vi "Day 9-2.vi"() -> ()   [LabVIEW 2019, in "Day 9.lvlib"]
uses:
  Day 9.lvlib
panel:
  out "result":i32
  out "Array 4":i32[](array[numeric])
  out "logical OR":bool
  out "Array 3":i32[][](array[numeric])
  out "x = y?":bool[][](array[boolean])
  out "Array":i32[][](array[numeric])
  in  "String":string="8969799987646798965432975435334567987976999867976794468999979759865767896545699865678952123899325456\n7658678998434597654321984320123458976765789998965432367998968998754556789434987654489543535698912349\n6243457899325679997620195431934569765654667999993101246796856997643245679759865443356954656987894498\n4102345678912998789531297659895978954213456899874512659965239876432134578998754321267899877976789987\n3212466989109887678942989797659799542102345798765423867894103987543026799989866532345678999765469896\n43234878932997954898999789879476896542434967898768649889432124986541359999679877654667899876543..."
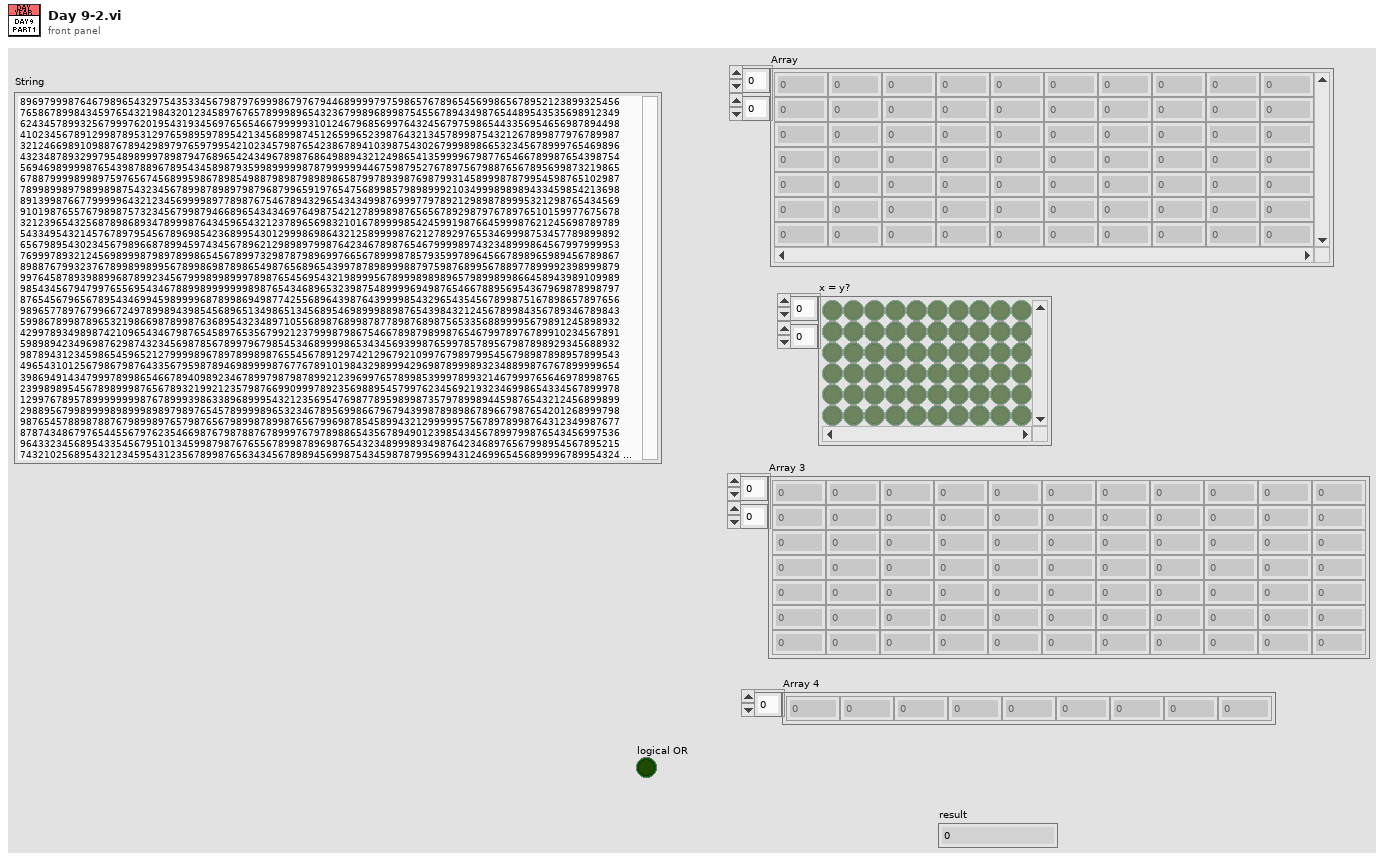
[diagram p1: front panel]
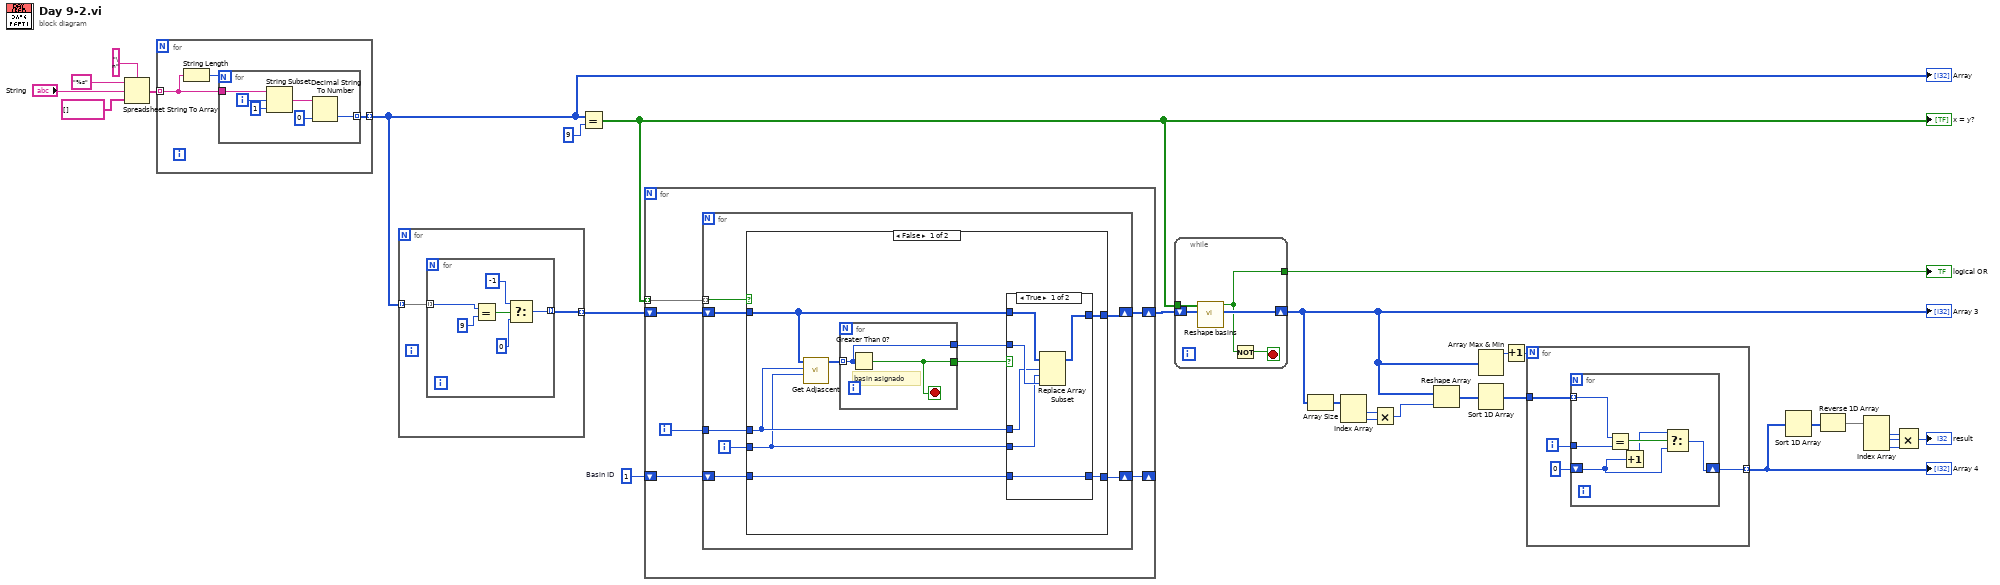
[diagram p0: block diagram]
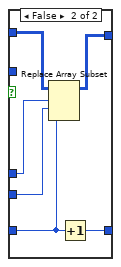
[diagram p2: hidden frame]
diagram:
  w22 = 1  # Basin ID
  n1 = Spreadsheet String To Array(delimiter (Tab)="\n", format string="%s", spreadsheet string="String", array type (2D Dbl)=string[] []) -> (array=w24:string[])
  n2 = for {
    tunnel: w24 -> [w31] mode=indexing
    tunnel: [w29] -> w21 mode=indexing
    n3 = String Length(string=w31) -> (length=w30:i32)
    n4 = for {
      N: w30 -> [_]
      tunnel: w31 -> [w37]
      tunnel: [w33] -> w29 mode=indexing
      i -> [w36]
      n5 = String Subset(string=w37, offset (0)=w36, length (rest)=1 ("length (rest)")) -> (substring=w34:string)
      n6 = Decimal String To Number(string=w34, default (0L)=0 ("default (0 I32)")) -> (number=w33:i32)  [unwired: 1 in, 1 out]
    }
  }
  "Array" <- w21
  n7 = for {
    tunnel: w21 -> [w39] mode=indexing
    tunnel: [w38] -> w20 mode=indexing
    n8 = for {
      tunnel: w39 -> [w44] mode=indexing
      tunnel: [w40] -> w38 mode=indexing
      n9 = Equal?(x=w44, y=9) -> (x = y?=w43:bool)
      n10 = Select(t=-1, s=w43, f=0) -> (s? t:f=w40:i32)
    }
  }
  n11 = Equal?(x=w21, y=9) -> (x = y?=w18:bool[][])
  "x = y?" <- w18
  n12 = for {
    tunnel: w18 -> [w51] mode=indexing
    shift-right: [w46] -> _
    shift-left: w22 -> [w49]
    shift-right: [w47] -> w19
    shift-left: w20 -> [w48]
    i -> [w50]
    n13 = for {
      tunnel: w51 -> [w58] mode=indexing
      tunnel: w50 -> [w56]
      shift-right: [w52] -> w46
      shift-left: w49 -> [w53]
      shift-right: [w54] -> w47
      shift-left: w48 -> [w57]
      i -> [w55]
      n14 = case shown="False" w58 {
        tunnel: w57 -> [w67 w82]
        tunnel: w56 -> [w63 _]
        tunnel: w55 -> [w62 _]
        tunnel: [w61 w82] -> w54
        tunnel: w53 -> [w60 w83]
        tunnel: [w59 w83] -> w52
        frame False {
          n15 = call "Get Adjascent.vi"("column"=w62, "row"=w63, "Array in"=w67) -> ("Array out"=w66:i32[])  [unwired: 8 in]
          n16 = for {
            tunnel: w66 -> [w69] mode=indexing
            tunnel: [w69] -> w64
            tunnel: [w68] -> w65
            stop <- w68 stop-if-true
            # "basin asignado"
            n17 = Greater Than 0?(x=w69) -> (x > 0?=w68:bool)
          }
          n18 = case shown="True" w65 {
            tunnel: w67 -> [w75 w81]
            tunnel: w64 -> [w74 _]
            tunnel: w63 -> [w73 w80]
            tunnel: w62 -> [w72 w79]
            tunnel: [w71 w78] -> w61
            tunnel: w60 -> [w70 w77]
            tunnel: [w70 w76] -> w59
            frame True {
              n19 = Replace Array Subset(array=w75, new element=w74, index (row)=w73, index (col)=w72) -> (w71:i32[][])
            }
            frame False {
              n20 = Replace Array Subset(array=w81, new element=w77, index (row)=w80, index (col)=w79) -> (w78:i32[][])
              n21 = Increment(x=w77) -> (x+1=w76:i32)
            }
          }
        }
        frame True {
        }
      }
    }
  }
  n22 = while {
    tunnel: w18 -> [w87]
    tunnel: [w85] -> w17
    shift-right: [w86] -> w12
    shift-left: w19 -> [w88]
    stop <- w84 stop-if-true
    n23 = call "Reshape basins.vi"("Array 3"=w88, "Array in"=w87) -> ("Array out"=w86:i32[][], "Boolean"=w85:bool)  [unwired: 8 in]
    n24 = Not(x=w85) -> (.not. x?=w84:bool)
  }
  "Array 3" <- w12
  "logical OR" <- w17
  n25 = Array Size(array=w12) -> (size(s)=w11:i32[])
  n26 = Index Array(array=w11) -> (element #1=w10:i32, element #2=w9:i32)  [unwired: 2 in]
  n27 = Multiply(x=w10, y=w9) -> (x*y=w8:i32)
  n28 = Reshape Array(w12, w8) -> (w16:i32[])
  n29 = Array Max & Min(array=w12) -> (max value=w13:i32)  [unwired: 3 out]
  n30 = Sort 1D Array(array=w16) -> (sorted array=w15:i32[])
  n31 = Increment(x=w13) -> (x+1=w14:i32)
  n32 = for {
    N: w14 -> [_]
    tunnel: w15 -> [w92]
    tunnel: [w89] -> w7 mode=indexing
    i -> [w91]
    n33 = for {
      tunnel: w92 -> [w98] mode=indexing
      tunnel: w91 -> [w97]
      shift-right: [w93] -> w89
      shift-left: 0 ("Basin ID") -> [w94]
      n34 = Equal?(x=w98, y=w97) -> (x = y?=w96:bool)
      n35 = Increment(x=w94) -> (x+1=w95:i32)
      n36 = Select(t=w95, s=w96, f=w94) -> (s? t:f=w93:i32)
    }
  }
  "Array 4" <- w7
  n37 = Sort 1D Array(array=w7) -> (sorted array=w6:i32[])
  n38 = Reverse 1D Array(array=w6) -> (reversed array=w5:i32[])
  n39 = Index Array(array=w5) -> (element #1=w4:i32, element #2=w3:i32, element #3=w2:i32)  [unwired: 3 in]
  n40 = Compound Arithmetic op=MULTIPLY(w4, w3, w2) -> (→"result":i32)
